vi "fmt_resetFormatBuffer.vi"(8 "error in (no error)":errorcluster, 11 "Format buffers in":T1) -> (0 "error out":errorcluster, 3 "Format buffers out":T1)   [LabVIEW 2017, in "NI_ExcelFile.lvlib"]
uses:
  <vilib>/express/express shared/NI_ExcelFile/NI_ExcelFile.lvlib
  <vilib>/express/express shared/NI_ExcelFile/Ctrls/fmt_formatBuffer.ctl
  <vilib>/express/express shared/NI_ExcelFile/Ctrls/TimeColumnMode.ctl
  <vilib>/express/express shared/NI_ExcelFile/Ctrls/Columns.ctl
  <vilib>/express/express shared/NI_ExcelFile/Ctrls/ColumnInfo.ctl
  <vilib>/express/express shared/NI_ExcelFile/Ctrls/DataType.ctl
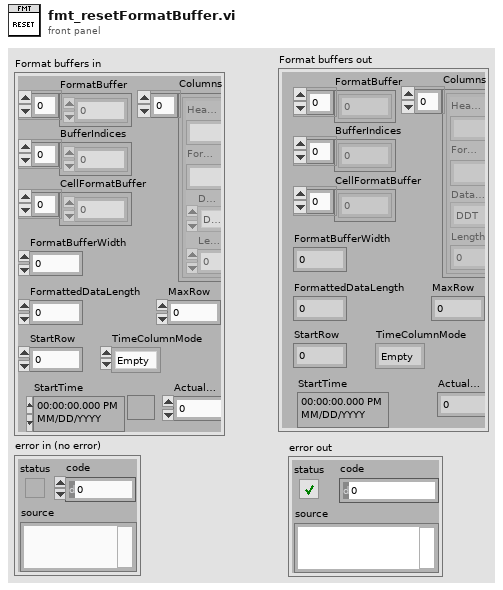
[diagram p1: front panel]
types:
  T1 = typedef "NI_ExcelFile.lvlib/fmt_formatBuffer.ctl" = cluster{"FormatBuffer":u8[], "BufferIndices":i32[], "CellFormatBuffer":u8[], "FormatBufferWidth":i32, "FormattedDataLength":i32, "MaxRow":i32, "StartRow":i32, "TimeColumnMode":T2, "StartTime":timestamp, "Columns":T3, "ActualLength":i32}
  T2 = typedef "NI_ExcelFile.lvlib/TimeColumnMode.ctl" = enum16{"Empty", "OnePerCh", "One"}
  T3 = typedef "NI_ExcelFile.lvlib/Columns.ctl" = T4[]
  T4 = typedef "NI_ExcelFile.lvlib/ColumnInfo.ctl" = cluster{"Header":string, "Format":string, "DataType":T5, "Length":u64}
  T5 = typedef "NI_ExcelFile.lvlib/DataType.ctl" = enum16{"DDT", "WFM", "Array of STR", "Array of DBL", "Array of I8", "Array of I16", "Array of I32", "Array of I64", "Array of SGL", "Array of U8", "Array of U16", "Array of U32", "Array of U64", "Array of Time"}
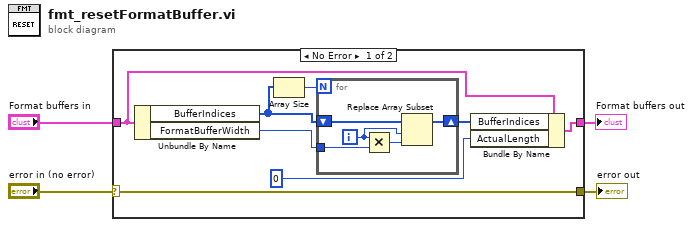
[diagram p0: block diagram]
diagram:
  n1 = case shown="No Error" "error in (no error)" {
    selector: "error in (no error)" -> [w6 w19]
    tunnel: [w12 w18] -> w4
    tunnel: "Format buffers in" -> [w11 w18]
    tunnel: [w6 w19] -> w1
    frame No Error {
      n2 = Unbundle By Name(w11) -> ("BufferIndices"=w7:i32[], "FormatBufferWidth"=w9:i32)
      n3 = Array Size(array=w7) -> (size(s)=w8:i32)
      n4 = for {
        N: w8 -> [_]
        tunnel: w9 -> [w13]
        shift-right: [w16] -> w10
        shift-left: w7 -> [w17]
        i -> [w14]
        n5 = Multiply(x=w14, y=w13) -> (x*y=w15:i32)
        n6 = Replace Array Subset(array=w17, new element=w15, index=w14) -> (w16:i32[])
      }
      n7 = Bundle By Name(cluster=w11, "BufferIndices"=w10, "ActualLength"=0) -> (w12:T1)
    }
    frame Error {
    }
  }
  "Format buffers out" <- w4
  "error out" <- w1
